vi "DL-Build.vi"() -> ()   [LabVIEW 2020]
panel:
  in  "Version":string="1.0"
  out "Progress Bar":u8(slide) caption="Finished!" scale=0.0..2.0
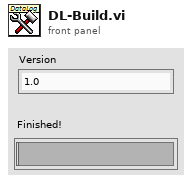
[diagram p1: front panel]
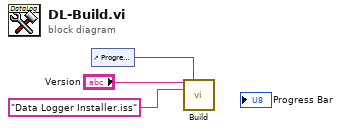
[diagram p0: block diagram]
diagram:
  n1 = control-ref of="Progress Bar"() -> (w2:refnum<vi>)
  n2 = call "Build.vi"("version"="Version", "Progress Bar"=w2, "iss path"="Data Logger Installer.iss") -> ()  [unwired: 13 in]
